vi "Notifier-with-memory-refnum.vi"(8 "error in":errorcluster, 10 "Timeout [ms]":i32, 11 "Notifier in":refnum<notifier>) -> (0 "error IO":errorcluster, 2 "Notification":enum16{""}(ring))   [LabVIEW 2013, in "CameraVision.lvlib" / "CV-UI.lvclass"]
uses:
  CV-UI.lvclass
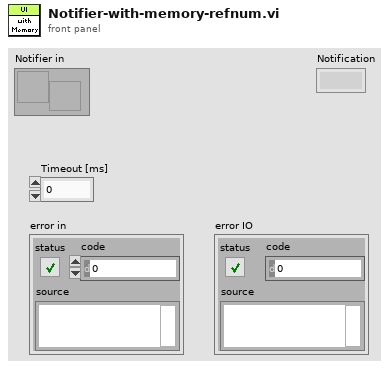
[diagram p1: front panel]
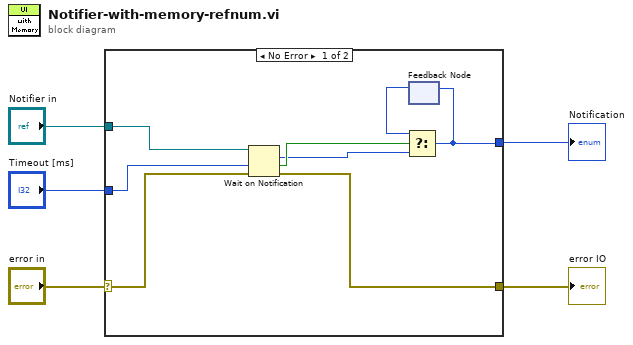
[diagram p0: block diagram]
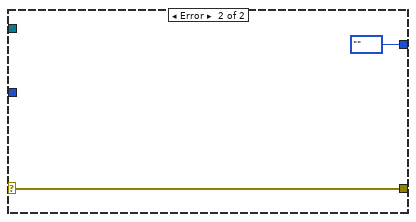
[diagram p2: hidden frame]
diagram:
  n1 = case shown="No Error" "error in" {
    selector: "error in" -> [w6 w14]
    tunnel: [w13 w14] -> w5
    tunnel: "Timeout [ms]" -> [w12 _]
    tunnel: "Notifier in" -> [w8 _]
    tunnel: [w7 enum16{""}.""] -> w2
    frame No Error {
      n2 = Wait on Notification(notifier=w8, timeout in ms (-1)=w12, error in (no error)=w6) -> (notification=w10:enum16{""}, timed out?=w11:bool, error out=w13:errorcluster)  [unwired: 1 in, 1 out]
      n3 = feedback #1() -> (w9:enum16{""})  [unwired: 1 in]
      n4 = Select(t=w9, s=w11, f=w10) -> (s? t:f=w7:enum16{""})
      n5 = feedback-in #1(w7) -> ()
    }
    frame Error {
    }
  }
  "error IO" <- w5
  "Notification" <- w2
